vi "Read Calibrations.vi"   [LabVIEW 2016]
uses:
  Global Variables/Deadband Calibrations.vi
  Global Variables/Turn to Heading Calibrations.vi
  Global Variables/Conveyor Calibrations.vi
  Global Variables/Shooter Calibrations.vi
  Global Variables/Ball Intake Calibrations.vi
  Global Variables/Drive Path Calibrations.vi
  Global Variables/Low Gear Calibrations.vi
  Global Variables/High Gear Calibrations.vi
  Global Variables/Auto Drive Calibrations.vi
  <vilib>/Rock Robotics/Network Tables/NT Write Numeric Array.vi
  <vilib>/Rock Robotics/Network Tables/NT Write Boolean.vi
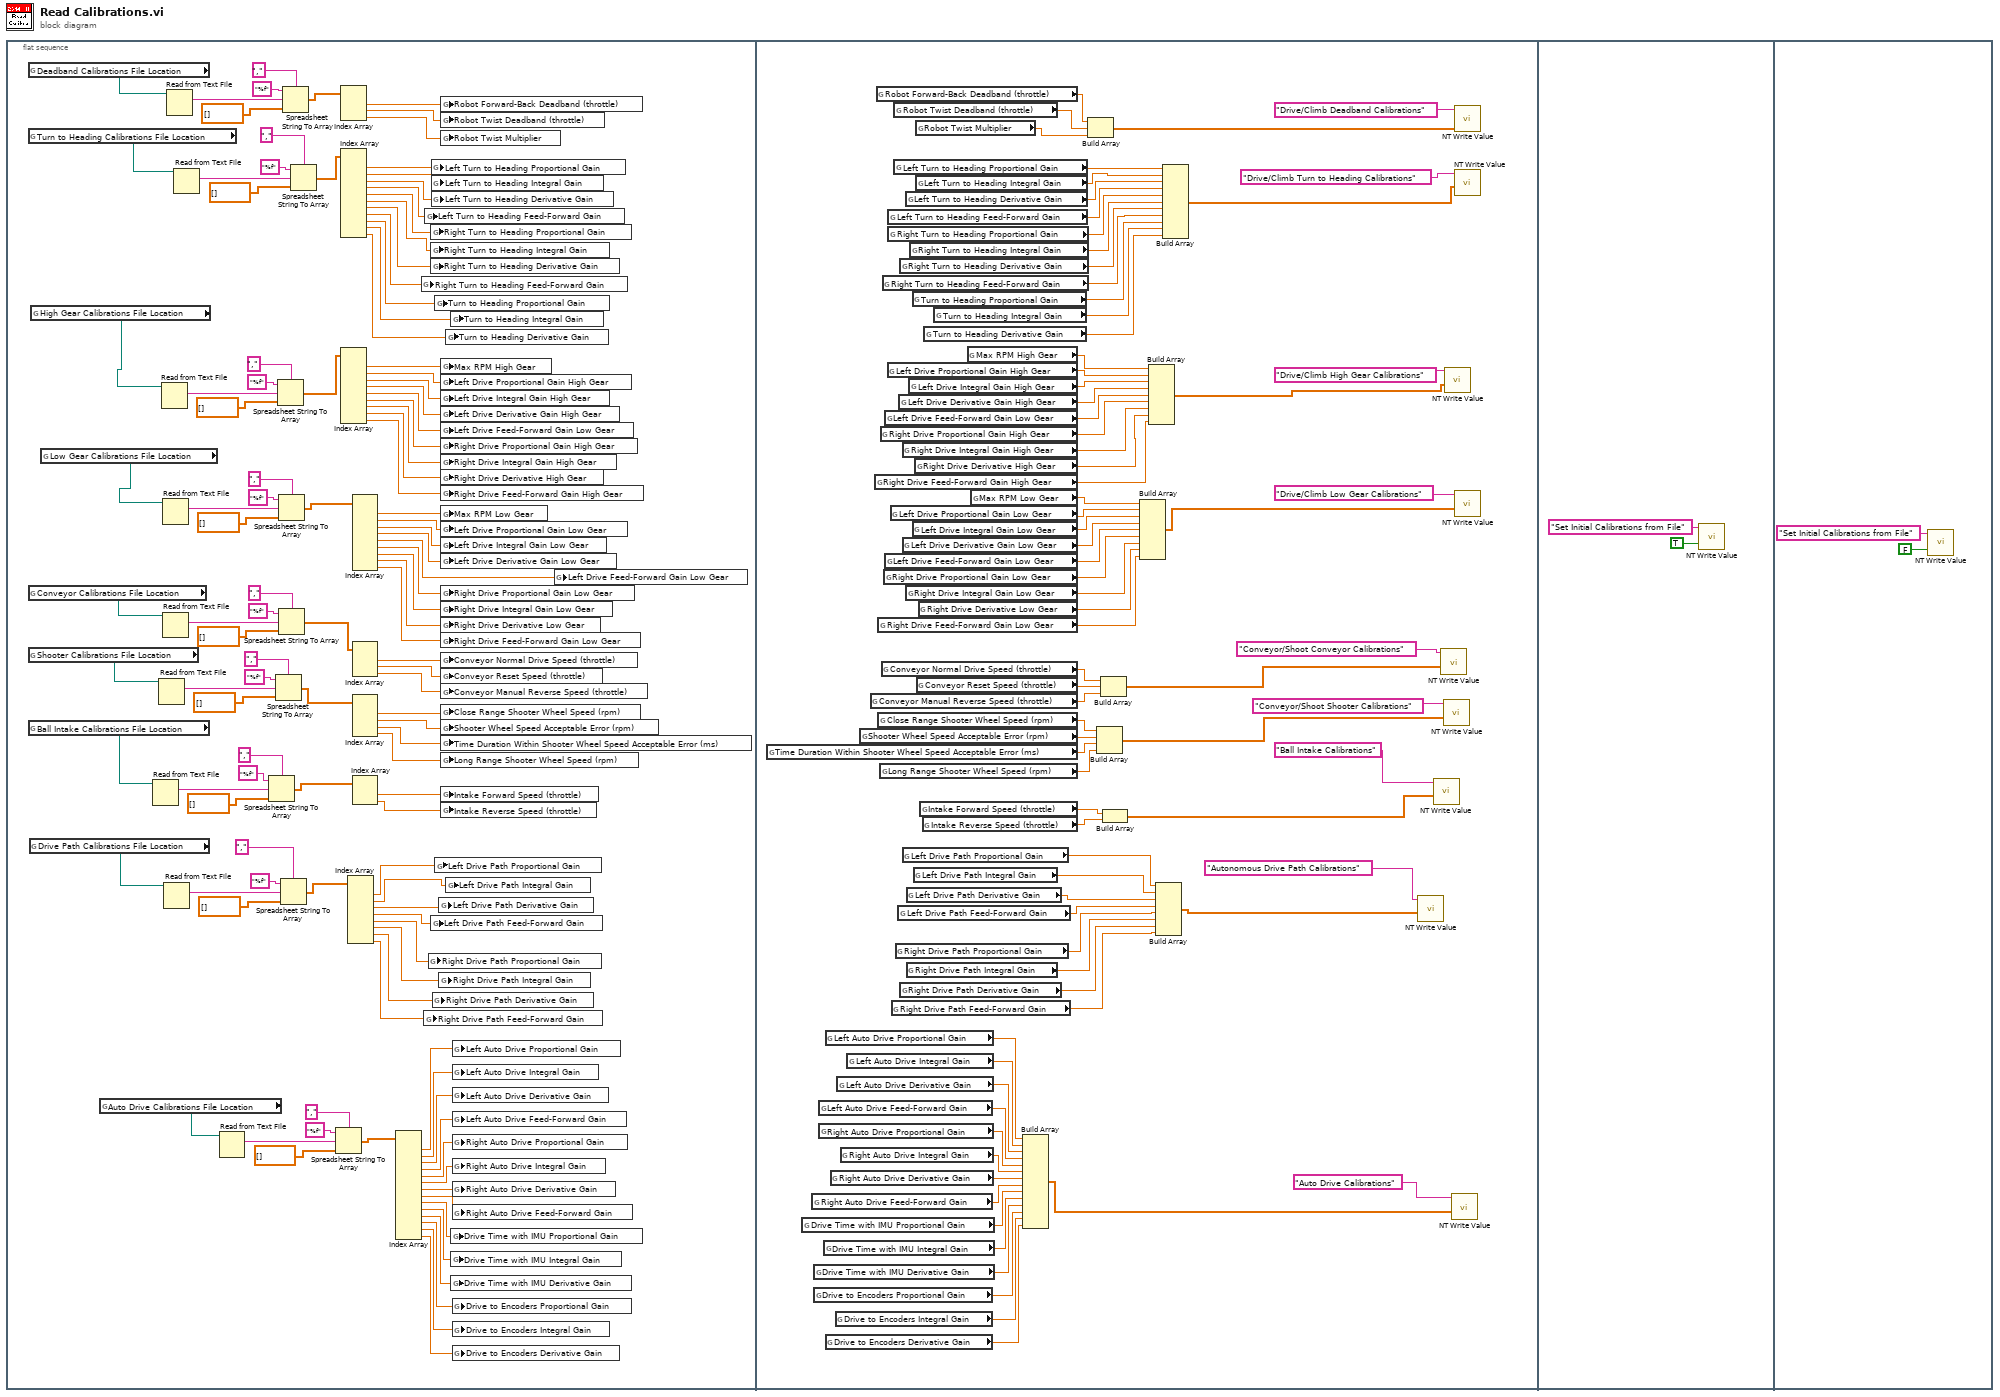
[diagram p0: block diagram]
diagram:
  n1 = flat-sequence {
    frame #0 {
      n2 = global read "Deadband Calibrations.vi" "Deadband Calibrations File Location"() -> (w110:path)
      n3 = global read "Turn to Heading Calibrations.vi" "Turn to Heading Calibrations File Location"() -> (w109:path)
      n4 = global read "Conveyor Calibrations.vi" "Conveyor Calibrations File Location"() -> (w88:path)
      n5 = global read "Shooter Calibrations.vi" "Shooter Calibrations File Location"() -> (w87:path)
      n6 = global read "Ball Intake Calibrations.vi" "Ball Intake Calibrations File Location"() -> (w86:path)
      n7 = global read "Drive Path Calibrations.vi" "Drive Path Calibrations File Location"() -> (w38:path)
      n8 = global read "High Gear Calibrations.vi" "High Gear Calibrations File Location"() -> (w27:path)
      n9 = global read "Low Gear Calibrations.vi" "Low Gear Calibrations File Location"() -> (w26:path)
      n10 = global read "Auto Drive Calibrations.vi" "Auto Drive Calibrations File Location"() -> (w16:path)
      n11 = Read from Text File(file (use dialog)=w86) -> (text=w92:string)  [unwired: 3 in, 3 out]
      n12 = Read from Text File(file (use dialog)=w87) -> (text=w96:string)  [unwired: 3 in, 3 out]
      n13 = Read from Text File(file (use dialog)=w27) -> (text=w108:string)  [unwired: 3 in, 3 out]
      n14 = Read from Text File(file (use dialog)=w26) -> (text=w104:string)  [unwired: 3 in, 3 out]
      n15 = Read from Text File(file (use dialog)=w88) -> (text=w100:string)  [unwired: 3 in, 3 out]
      n16 = Read from Text File(file (use dialog)=w38) -> (text=w39:string)  [unwired: 3 in, 3 out]
      n17 = Read from Text File(file (use dialog)=w110) -> (text=w114:string)  [unwired: 3 in, 3 out]
      n18 = Read from Text File(file (use dialog)=w109) -> (text=w117:string)  [unwired: 3 in, 3 out]
      n19 = Read from Text File(file (use dialog)=w16) -> (text=w20:string)  [unwired: 3 in, 3 out]
      n20 = Spreadsheet String To Array(delimiter (Tab)=",", format string="%f", spreadsheet string=w92, array type (2D Dbl)=dbl[] []) -> (array=w47:dbl[])
      n21 = Spreadsheet String To Array(delimiter (Tab)=",", format string="%f", spreadsheet string=w96, array type (2D Dbl)=dbl[] []) -> (array=w48:dbl[])
      n22 = Spreadsheet String To Array(delimiter (Tab)=",", format string="%f", spreadsheet string=w108, array type (2D Dbl)=dbl[] []) -> (array=w51:dbl[])
      n23 = Spreadsheet String To Array(delimiter (Tab)=",", format string="%f", spreadsheet string=w104, array type (2D Dbl)=dbl[] []) -> (array=w50:dbl[])
      n24 = Spreadsheet String To Array(delimiter (Tab)=",", format string="%f", spreadsheet string=w100, array type (2D Dbl)=dbl[] []) -> (array=w49:dbl[])
      n25 = Spreadsheet String To Array(delimiter (Tab)=",", format string="%f", spreadsheet string=w39, array type (2D Dbl)=dbl[] []) -> (array=w36:dbl[])
      n26 = Spreadsheet String To Array(delimiter (Tab)=",", format string="%f", spreadsheet string=w114, array type (2D Dbl)=dbl[] []) -> (array=w53:dbl[])
      n27 = Spreadsheet String To Array(delimiter (Tab)=",", format string="%f", spreadsheet string=w117, array type (2D Dbl)=dbl[] []) -> (array=w52:dbl[])
      n28 = Spreadsheet String To Array(delimiter (Tab)=",", format string="%f", spreadsheet string=w20, array type (2D Dbl)=dbl[] []) -> (array=w1:dbl[])
      n29 = Index Array(array=w53) -> (element #1=w84:dbl, element #2=w83:dbl, element #3=w21:dbl)  [unwired: 3 in]
      n30 = Index Array(array=w52) -> (element #1=w76:dbl, element #2=w75:dbl, element #3=w74:dbl, element #4=w46:dbl, element #5=w45:dbl, element #6=w44:dbl, element #7=w43:dbl, element #8=w42:dbl, element #9=w24:dbl, element #10=w23:dbl, element #11=w22:dbl)  [unwired: 11 in]
      n31 = Index Array(array=w51) -> (element #1=w77:dbl, element #2=w73:dbl, element #3=w72:dbl, element #4=w71:dbl, element #5=w70:dbl, element #6=w69:dbl, element #7=w68:dbl, element #8=w67:dbl, element #9=w66:dbl)  [unwired: 9 in]
      n32 = Index Array(array=w36) -> (element #1=w35:dbl, element #2=w34:dbl, element #3=w33:dbl, element #4=w32:dbl, element #5=w31:dbl, element #6=w28:dbl, element #7=w29:dbl, element #8=w30:dbl)  [unwired: 8 in]
      n33 = Index Array(array=w50) -> (element #1=w78:dbl, element #2=w65:dbl, element #3=w64:dbl, element #4=w63:dbl, element #5=w62:dbl, element #6=w61:dbl, element #7=w60:dbl, element #8=w59:dbl, element #9=w58:dbl)  [unwired: 9 in]
      n34 = Index Array(array=w49) -> (element #1=w57:dbl, element #2=w56:dbl, element #3=w79:dbl)  [unwired: 3 in]
      n35 = Index Array(array=w48) -> (element #1=w81:dbl, element #2=w55:dbl, element #3=w80:dbl, element #4=w25:dbl)  [unwired: 4 in]
      n36 = Index Array(array=w47) -> (element #1=w82:dbl, element #2=w54:dbl)  [unwired: 2 in]
      n37 = Index Array(array=w1) -> (element #1=w15:dbl, element #2=w14:dbl, element #3=w13:dbl, element #4=w12:dbl, element #5=w11:dbl, element #6=w10:dbl, element #7=w9:dbl, element #8=w8:dbl, element #9=w7:dbl, element #10=w6:dbl, element #11=w5:dbl, element #12=w4:dbl, element #13=w3:dbl, element #14=w2:dbl)  [unwired: 14 in]
      n38 = global write "Turn to Heading Calibrations.vi" "Right Turn to Heading Feed-Forward Gain"(w42) -> ()
      n39 = global write "Drive Path Calibrations.vi" "Right Drive Path Feed-Forward Gain"(w30) -> ()
      n40 = global write "Turn to Heading Calibrations.vi" "Left Turn to Heading Feed-Forward Gain"(w46) -> ()
      n41 = global write "Drive Path Calibrations.vi" "Right Drive Path Proportional Gain"(w31) -> ()
      n42 = global write "Turn to Heading Calibrations.vi" "Right Turn to Heading Proportional Gain"(w45) -> ()
      n43 = global write "Turn to Heading Calibrations.vi" "Right Turn to Heading Integral Gain"(w44) -> ()
      n44 = global write "Turn to Heading Calibrations.vi" "Right Turn to Heading Derivative Gain"(w43) -> ()
      n45 = global write "Drive Path Calibrations.vi" "Left Drive Path Feed-Forward Gain"(w32) -> ()
      n46 = global write "Turn to Heading Calibrations.vi" "Left Turn to Heading Proportional Gain"(w76) -> ()
      n47 = global write "Turn to Heading Calibrations.vi" "Left Turn to Heading Integral Gain"(w75) -> ()
      n48 = global write "Turn to Heading Calibrations.vi" "Left Turn to Heading Derivative Gain"(w74) -> ()
      n49 = global write "Drive Path Calibrations.vi" "Right Drive Path Derivative Gain"(w29) -> ()
      n50 = global write "Turn to Heading Calibrations.vi" "Turn to Heading Proportional Gain"(w24) -> ()
      n51 = global write "Drive Path Calibrations.vi" "Left Drive Path Proportional Gain"(w35) -> ()
      n52 = global write "Drive Path Calibrations.vi" "Left Drive Path Derivative Gain"(w33) -> ()
      n53 = global write "Drive Path Calibrations.vi" "Right Drive Path Integral Gain"(w28) -> ()
      n54 = global write "Deadband Calibrations.vi" "Robot Forward-Back Deadband (throttle)"(w84) -> ()
      n55 = global write "Deadband Calibrations.vi" "Robot Twist Deadband (throttle)"(w83) -> ()
      n56 = global write "Deadband Calibrations.vi" "Robot Twist Multiplier"(w21) -> ()
      n57 = global write "High Gear Calibrations.vi" "Max RPM High Gear"(w77) -> ()
      n58 = global write "High Gear Calibrations.vi" "Left Drive Proportional Gain High Gear"(w73) -> ()
      n59 = global write "High Gear Calibrations.vi" "Left Drive Integral Gain High Gear"(w72) -> ()
      n60 = global write "High Gear Calibrations.vi" "Left Drive Derivative Gain High Gear"(w71) -> ()
      n61 = global write "High Gear Calibrations.vi" "Left Drive Feed-Forward Gain Low Gear"(w70) -> ()
      n62 = global write "High Gear Calibrations.vi" "Right Drive Proportional Gain High Gear"(w69) -> ()
      n63 = global write "High Gear Calibrations.vi" "Right Drive Integral Gain High Gear"(w68) -> ()
      n64 = global write "High Gear Calibrations.vi" "Right Drive Derivative High Gear"(w67) -> ()
      n65 = global write "High Gear Calibrations.vi" "Right Drive Feed-Forward Gain High Gear"(w66) -> ()
      n66 = global write "Low Gear Calibrations.vi" "Max RPM Low Gear"(w78) -> ()
      n67 = global write "Low Gear Calibrations.vi" "Left Drive Proportional Gain Low Gear"(w65) -> ()
      n68 = global write "Low Gear Calibrations.vi" "Left Drive Integral Gain Low Gear"(w64) -> ()
      n69 = global write "Low Gear Calibrations.vi" "Left Drive Derivative Gain Low Gear"(w63) -> ()
      n70 = global write "Low Gear Calibrations.vi" "Right Drive Proportional Gain Low Gear"(w61) -> ()
      n71 = global write "Low Gear Calibrations.vi" "Right Drive Integral Gain Low Gear"(w60) -> ()
      n72 = global write "Low Gear Calibrations.vi" "Right Drive Derivative Low Gear"(w59) -> ()
      n73 = global write "Low Gear Calibrations.vi" "Right Drive Feed-Forward Gain Low Gear"(w58) -> ()
      n74 = global write "Conveyor Calibrations.vi" "Conveyor Normal Drive Speed (throttle)"(w57) -> ()
      n75 = global write "Conveyor Calibrations.vi" "Conveyor Reset Speed (throttle)"(w56) -> ()
      n76 = global write "Conveyor Calibrations.vi" "Conveyor Manual Reverse Speed (throttle)"(w79) -> ()
      n77 = global write "Shooter Calibrations.vi" "Close Range Shooter Wheel Speed (rpm)"(w81) -> ()
      n78 = global write "Shooter Calibrations.vi" "Shooter Wheel Speed Acceptable Error (rpm)"(w55) -> ()
      n79 = global write "Shooter Calibrations.vi" "Time Duration Within Shooter Wheel Speed Acceptable Error (ms)"(w80) -> ()
      n80 = global write "Shooter Calibrations.vi" "Long Range Shooter Wheel Speed (rpm)"(w25) -> ()
      n81 = global write "Ball Intake Calibrations.vi" "Intake Forward Speed (throttle)"(w82) -> ()
      n82 = global write "Ball Intake Calibrations.vi" "Intake Reverse Speed (throttle)"(w54) -> ()
      n83 = global write "Turn to Heading Calibrations.vi" "Turn to Heading Derivative Gain"(w22) -> ()
      n84 = global write "Drive Path Calibrations.vi" "Left Drive Path Integral Gain"(w34) -> ()
      n85 = global write "Turn to Heading Calibrations.vi" "Turn to Heading Integral Gain"(w23) -> ()
      n86 = global write "Auto Drive Calibrations.vi" "Drive Time with IMU Proportional Gain"(w7) -> ()
      n87 = global write "Auto Drive Calibrations.vi" "Drive Time with IMU Integral Gain"(w6) -> ()
      n88 = global write "Auto Drive Calibrations.vi" "Drive Time with IMU Derivative Gain"(w5) -> ()
      n89 = global write "Auto Drive Calibrations.vi" "Left Auto Drive Proportional Gain"(w15) -> ()
      n90 = global write "Auto Drive Calibrations.vi" "Left Auto Drive Integral Gain"(w14) -> ()
      n91 = global write "Auto Drive Calibrations.vi" "Left Auto Drive Derivative Gain"(w13) -> ()
      n92 = global write "Auto Drive Calibrations.vi" "Left Auto Drive Feed-Forward Gain"(w12) -> ()
      n93 = global write "Auto Drive Calibrations.vi" "Right Auto Drive Proportional Gain"(w11) -> ()
      n94 = global write "Auto Drive Calibrations.vi" "Right Auto Drive Integral Gain"(w10) -> ()
      n95 = global write "Auto Drive Calibrations.vi" "Right Auto Drive Derivative Gain"(w9) -> ()
      n96 = global write "Auto Drive Calibrations.vi" "Right Auto Drive Feed-Forward Gain"(w8) -> ()
      n97 = global write "Auto Drive Calibrations.vi" "Drive to Encoders Proportional Gain"(w4) -> ()
      n98 = global write "Auto Drive Calibrations.vi" "Drive to Encoders Integral Gain"(w3) -> ()
      n99 = global write "Auto Drive Calibrations.vi" "Drive to Encoders Derivative Gain"(w2) -> ()
      n100 = global write "Low Gear Calibrations.vi" "Left Drive Feed-Forward Gain Low Gear"(w62) -> ()
    }
    frame #1 {
      n101 = global read "Shooter Calibrations.vi" "Time Duration Within Shooter Wheel Speed Acceptable Error (ms)"() -> (w170:dbl)
      n102 = global read "Auto Drive Calibrations.vi" "Drive Time with IMU Proportional Gain"() -> (w125:dbl)
      n103 = global read "Auto Drive Calibrations.vi" "Right Auto Drive Feed-Forward Gain"() -> (w126:dbl)
      n104 = global read "Auto Drive Calibrations.vi" "Drive Time with IMU Derivative Gain"() -> (w123:dbl)
      n105 = global read "Auto Drive Calibrations.vi" "Drive to Encoders Proportional Gain"() -> (w122:dbl)
      n106 = global read "Auto Drive Calibrations.vi" "Left Auto Drive Feed-Forward Gain"() -> (w130:dbl)
      n107 = global read "Auto Drive Calibrations.vi" "Right Auto Drive Proportional Gain"() -> (w129:dbl)
      n108 = global read "Auto Drive Calibrations.vi" "Drive Time with IMU Integral Gain"() -> (w124:dbl)
      n109 = global read "Auto Drive Calibrations.vi" "Left Auto Drive Proportional Gain"() -> (w133:dbl)
      n110 = global read "Auto Drive Calibrations.vi" "Drive to Encoders Derivative Gain"() -> (w120:dbl)
      n111 = global read "Auto Drive Calibrations.vi" "Right Auto Drive Derivative Gain"() -> (w127:dbl)
      n112 = global read "Auto Drive Calibrations.vi" "Drive to Encoders Integral Gain"() -> (w121:dbl)
      n113 = global read "Auto Drive Calibrations.vi" "Left Auto Drive Derivative Gain"() -> (w131:dbl)
      n114 = global read "Auto Drive Calibrations.vi" "Right Auto Drive Integral Gain"() -> (w128:dbl)
      n115 = global read "Auto Drive Calibrations.vi" "Left Auto Drive Integral Gain"() -> (w132:dbl)
      n116 = global read "Shooter Calibrations.vi" "Shooter Wheel Speed Acceptable Error (rpm)"() -> (w171:dbl)
      n117 = global read "Conveyor Calibrations.vi" "Conveyor Manual Reverse Speed (throttle)"() -> (w172:dbl)
      n118 = global read "High Gear Calibrations.vi" "Right Drive Feed-Forward Gain High Gear"() -> (w183:dbl)
      n119 = global read "Deadband Calibrations.vi" "Robot Forward-Back Deadband (throttle)"() -> (w192:dbl)
      n120 = global read "Low Gear Calibrations.vi" "Right Drive Feed-Forward Gain Low Gear"() -> (w167:dbl)
      n121 = global read "Shooter Calibrations.vi" "Close Range Shooter Wheel Speed (rpm)"() -> (w140:dbl)
      n122 = global read "Shooter Calibrations.vi" "Long Range Shooter Wheel Speed (rpm)"() -> (w139:dbl)
      n123 = global read "High Gear Calibrations.vi" "Right Drive Proportional Gain High Gear"() -> (w186:dbl)
      n124 = global read "Conveyor Calibrations.vi" "Conveyor Normal Drive Speed (throttle)"() -> (w174:dbl)
      n125 = global read "Turn to Heading Calibrations.vi" "Right Turn to Heading Feed-Forward Gain"() -> (w152:dbl)
      n126 = global read "Low Gear Calibrations.vi" "Right Drive Proportional Gain Low Gear"() -> (w177:dbl)
      n127 = global read "High Gear Calibrations.vi" "Left Drive Feed-Forward Gain Low Gear"() -> (w187:dbl)
      n128 = global read "Low Gear Calibrations.vi" "Left Drive Feed-Forward Gain Low Gear"() -> (w178:dbl)
      n129 = global read "High Gear Calibrations.vi" "Left Drive Proportional Gain High Gear"() -> (w190:dbl)
      n130 = global read "Turn to Heading Calibrations.vi" "Left Turn to Heading Feed-Forward Gain"() -> (w156:dbl)
      n131 = global read "Turn to Heading Calibrations.vi" "Right Turn to Heading Proportional Gain"() -> (w155:dbl)
      n132 = global read "Low Gear Calibrations.vi" "Left Drive Proportional Gain Low Gear"() -> (w181:dbl)
      n133 = global read "Drive Path Calibrations.vi" "Right Drive Path Feed-Forward Gain"() -> (w142:dbl)
      n134 = global read "Deadband Calibrations.vi" "Robot Twist Deadband (throttle)"() -> (w193:dbl)
      n135 = global read "Turn to Heading Calibrations.vi" "Left Turn to Heading Proportional Gain"() -> (w159:dbl)
      n136 = global read "Drive Path Calibrations.vi" "Right Drive Path Proportional Gain"() -> (w145:dbl)
      n137 = global read "Drive Path Calibrations.vi" "Left Drive Path Feed-Forward Gain"() -> (w146:dbl)
      n138 = global read "High Gear Calibrations.vi" "Left Drive Derivative Gain High Gear"() -> (w188:dbl)
      n139 = global read "Turn to Heading Calibrations.vi" "Right Turn to Heading Derivative Gain"() -> (w153:dbl)
      n140 = global read "Drive Path Calibrations.vi" "Right Drive Path Derivative Gain"() -> (w143:dbl)
      n141 = global read "High Gear Calibrations.vi" "Right Drive Integral Gain High Gear"() -> (w185:dbl)
      n142 = global read "Low Gear Calibrations.vi" "Left Drive Derivative Gain Low Gear"() -> (w179:dbl)
      n143 = global read "Drive Path Calibrations.vi" "Left Drive Path Proportional Gain"() -> (w149:dbl)
      n144 = global read "Turn to Heading Calibrations.vi" "Left Turn to Heading Derivative Gain"() -> (w157:dbl)
      n145 = global read "Low Gear Calibrations.vi" "Right Drive Integral Gain Low Gear"() -> (w176:dbl)
      n146 = global read "Drive Path Calibrations.vi" "Left Drive Path Derivative Gain"() -> (w147:dbl)
      n147 = global read "Drive Path Calibrations.vi" "Right Drive Path Integral Gain"() -> (w144:dbl)
      n148 = global read "High Gear Calibrations.vi" "Left Drive Integral Gain High Gear"() -> (w189:dbl)
      n149 = global read "Turn to Heading Calibrations.vi" "Right Turn to Heading Integral Gain"() -> (w154:dbl)
      n150 = global read "Turn to Heading Calibrations.vi" "Turn to Heading Proportional Gain"() -> (w138:dbl)
      n151 = global read "Low Gear Calibrations.vi" "Left Drive Integral Gain Low Gear"() -> (w180:dbl)
      n152 = global read "Drive Path Calibrations.vi" "Left Drive Path Integral Gain"() -> (w148:dbl)
      n153 = global read "High Gear Calibrations.vi" "Right Drive Derivative High Gear"() -> (w184:dbl)
      n154 = global read "Deadband Calibrations.vi" "Robot Twist Multiplier"() -> (w134:dbl)
      n155 = global read "Turn to Heading Calibrations.vi" "Left Turn to Heading Integral Gain"() -> (w158:dbl)
      n156 = global read "Conveyor Calibrations.vi" "Conveyor Reset Speed (throttle)"() -> (w173:dbl)
      n157 = global read "Low Gear Calibrations.vi" "Right Drive Derivative Low Gear"() -> (w175:dbl)
      n158 = global read "Ball Intake Calibrations.vi" "Intake Forward Speed (throttle)"() -> (w169:dbl)
      n159 = global read "Ball Intake Calibrations.vi" "Intake Reverse Speed (throttle)"() -> (w168:dbl)
      n160 = global read "Turn to Heading Calibrations.vi" "Turn to Heading Derivative Gain"() -> (w136:dbl)
      n161 = global read "Turn to Heading Calibrations.vi" "Turn to Heading Integral Gain"() -> (w137:dbl)
      n162 = global read "High Gear Calibrations.vi" "Max RPM High Gear"() -> (w191:dbl)
      n163 = global read "Low Gear Calibrations.vi" "Max RPM Low Gear"() -> (w182:dbl)
      n164 = Build Array(w133, w132, w131, w130, w129, w128, w127, w126, w125, w124, w123, w122, w121, w120) -> (w118:dbl[])
      n165 = Build Array(w192, w193, w134) -> (w166:dbl[])
      n166 = Build Array(w140, w171, w170, w139) -> (w162:dbl[])
      n167 = Build Array(w174, w173, w172) -> (w163:dbl[])
      n168 = Build Array(w169, w168) -> (w161:dbl[])
      n169 = Build Array(w182, w181, w180, w179, w178, w177, w176, w175, w167) -> (w164:dbl[])
      n170 = Build Array(w191, w190, w189, w188, w187, w186, w185, w184, w183) -> (w165:dbl[])
      n171 = Build Array(w149, w148, w147, w146, w145, w144, w143, w142) -> (w141:dbl[])
      n172 = Build Array(w159, w158, w157, w156, w155, w154, w153, w152, w138, w137, w136) -> (w151:dbl[])
      n173 = call-poly <vilib>:"NT Write Value.vi"("Numeric Array"=w141, "Name"="Autonomous Drive Path Calibrations") -> ()  [unwired: 9 in, 1 out]
      n174 = call-poly <vilib>:"NT Write Value.vi"("Numeric Array"=w161, "Name"="Ball Intake Calibrations") -> ()  [unwired: 9 in, 1 out]
      n175 = call-poly <vilib>:"NT Write Value.vi"("Numeric Array"=w163, "Name"="Conveyor/Shoot Conveyor Calibrations") -> ()  [unwired: 9 in, 1 out]
      n176 = call-poly <vilib>:"NT Write Value.vi"("Numeric Array"=w162, "Name"="Conveyor/Shoot Shooter Calibrations") -> ()  [unwired: 9 in, 1 out]
      n177 = call-poly <vilib>:"NT Write Value.vi"("Numeric Array"=w165, "Name"="Drive/Climb High Gear Calibrations") -> ()  [unwired: 9 in, 1 out]
      n178 = call-poly <vilib>:"NT Write Value.vi"("Numeric Array"=w118, "Name"="Auto Drive Calibrations") -> ()  [unwired: 9 in, 1 out]
      n179 = call-poly <vilib>:"NT Write Value.vi"("Numeric Array"=w166, "Name"="Drive/Climb Deadband Calibrations") -> ()  [unwired: 9 in, 1 out]
      n180 = call-poly <vilib>:"NT Write Value.vi"("Numeric Array"=w151, "Name"="Drive/Climb Turn to Heading Calibrations") -> ()  [unwired: 9 in, 1 out]
      n181 = call-poly <vilib>:"NT Write Value.vi"("Numeric Array"=w164, "Name"="Drive/Climb Low Gear Calibrations") -> ()  [unwired: 9 in, 1 out]
    }
    frame #2 {
      n182 = call-poly <vilib>:"NT Write Value.vi"("Boolean"=TRUE, "Name"="Set Initial Calibrations from File") -> ()  [unwired: 9 in, 1 out]
    }
    frame #3 {
      n183 = call-poly <vilib>:"NT Write Value.vi"("Boolean"=FALSE, "Name"="Set Initial Calibrations from File") -> ()  [unwired: 9 in, 1 out]
    }
  }
